vi "Logger.vi"() -> ()   [LabVIEW 2025]
uses:
  LOGmanager.vi
  LOGlib.lvlib
panel:
  in  "LOG file path (user Documents folder)":string="C:\\Users\\paillotte\\Documents\\LOG"
  in  "Error":bool
  in  "stop":bool
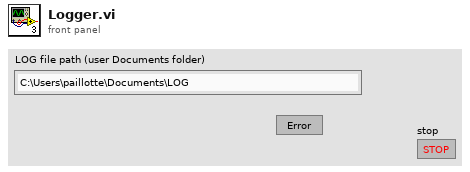
[diagram p1: front panel]
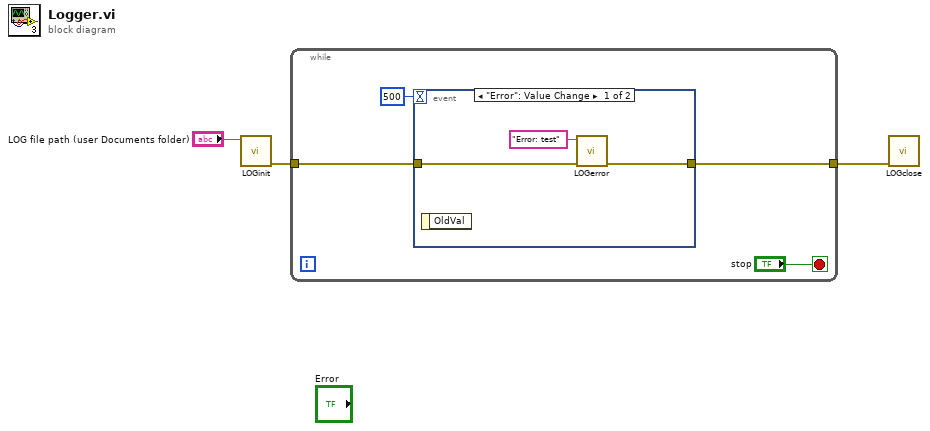
[diagram p0: block diagram]
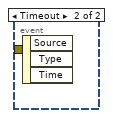
[diagram p2: hidden frame]
diagram:
  n1 = call "LOGinit.vi"("LOG file path (user Documents folder)"="LOG file path (user Documents folder)") -> ("error out"=w3:errorcluster)  [unwired: 10 in]
  n2 = while {
    tunnel: [w5] -> w2
    tunnel: w3 -> [w6]
    stop <- "stop" stop-if-true
    n3 = event shown="[0] \"Error\": Value Change" {
      selector: _ -> [_ _]
      dyn-events: _ -> [_ _]
      timeout: 500 -> [_ _]
      tunnel: w6 -> [w10 _]
      tunnel: [w9 _] -> w5
      event "Error": Value Change {
        n4 = event-data() -> ()  [unwired: 1 in, 1 out]
        n5 = call "LOGerror.vi"("Error In"=w10, "Message"="Error: test") -> ("Error Out"=w9:errorcluster)  [unwired: 9 in]
      }
      event Timeout {
        n6 = event-data() -> ()  [unwired: 1 in, 3 out]
      }
    }
  }
  n7 = call "LOGclose.vi"("error in (no error)"=w2) -> ()  [unwired: 11 in]
